vi "Read Severity.vi"(8 "error in":errorcluster, 11 "Has Alarm in":refnum<class "Has Alarm.lvclass">) -> (0 "error out":errorcluster, 2 "severity":T1, 3 "Has Alarm out":refnum<class "Has Alarm.lvclass">)   [LabVIEW 2020, in "PV Access.lvlib" / "PV Data.lvlib" / "Has Alarm.lvclass"]
uses:
  Has Alarm.lvclass
  182da66a-f6ee-47d3-9b05-9cecdf4c7a27.vi
  Alarm Severity.ctl
  PV Data.lvlib
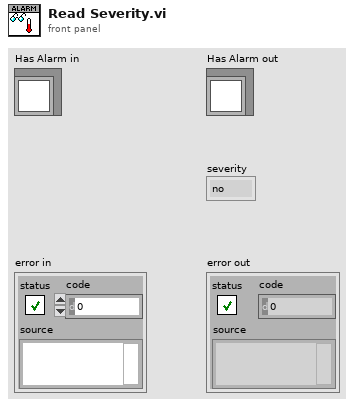
[diagram p1: front panel]
types:
  T1 = typedef "PV Access.lvlib/PV Data.lvlib/Alarm Severity.ctl" = enum32{"no", "minor", "major", "record", "invalid", "undefined"}
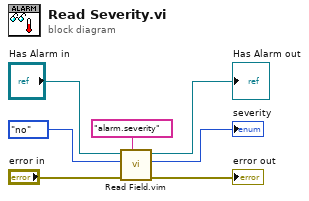
[diagram p0: block diagram]
diagram:
  n1 = call "Read Field.vim"("field"="alarm.severity" ("element name"), "error in"="error in", "default value"=Alarm_Severity."no" ("Severity"), "Base Interface in"="Has Alarm in") -> ("error out"=→"error out":errorcluster, "value"=→"severity":T1, "Base Interface out"=→"Has Alarm out":refnum<class "Has Alarm.lvclass">)  [unwired: 5 in]
